vi "KF 연습 (A=eye(2)).vi"(2 "R":dbl[][](array[numeric])=[[1e-05, 0.0], [0.0, 1e-05]], 3 "Q":dbl[][](array[numeric])=[[0.001, 0.0], [0.0, 0.001]], 4 "Y_input":dbl format="%#.8g", 5 "X_input":dbl format="%#.8g") -> (0 "Y_Filtered":dbl format="%#.8g", 1 "X_Filtered":dbl format="%#.8g")   [LabVIEW 2016]
uses:
  <vilib>/imath/engines/lvmath2/RunTimeEngine/IndexRead/NIMS M(S).vi
  <instcachedir>/0/NIMS M(S)_B826C018497E4940AE96BD27B540B6FB.lvgen/NIMS M(S)_B826C018497E4940AE96BD27B540B6FB_000.vi
  <vilib>/imathl/engines/lvmath/Functions/Error Handling/Create Error.vi
  <vilib>/imath/engines/lvmath2/RunTimeEngine/ArithmeticOperatorToken/NIMS_ArithmeticOperator_multmx.vi
  <instcachedir>/0/NIMS_ArithmeticOperator_multmx_4A56FE5C615140CE835D4DB5891BF065.lvgen/NIMS_ArithmeticOperator_multmx_4A56FE5C615140CE835D4DB5891BF065_005.vi
  <instcachedir>/0/NIMS_ArithmeticOperator_multmx_4A56FE5C615140CE835D4DB5891BF065.lvgen/NIMS_ArithmeticOperator_multmx_4A56FE5C615140CE835D4DB5891BF065_006.vi
  <vilib>/imath/engines/lvmath2/RunTimeEngine/ArithmeticOperatorToken/NIMS_ArithmeticOperator_plus.vi
  <instcachedir>/0/NIMS_ArithmeticOperator_plus_0120E0498A0F4B4B9BDCAC2554767A4E.lvgen/NIMS_ArithmeticOperator_plus_0120E0498A0F4B4B9BDCAC2554767A4E_003.vi
  <vilib>/imath/engines/lvmath2/RunTimeEngine/ErrorHandling/NIMS_Create Error From Enums.vi
  <vilib>/imath/engines/lvmath2/RunTimeEngine/BuiltInFunctions/inv/NIMS_inv(GM).vi
  <instcachedir>/0/NIMS_inv(GM)_A6DF8FE880224208AACFE4CF9F659502.lvgen/NIMS_inv(GM)_A6DF8FE880224208AACFE4CF9F659502_000.vi
  <instcachedir>/0/NIMS_ArithmeticOperator_multmx_4A56FE5C615140CE835D4DB5891BF065.lvgen/NIMS_ArithmeticOperator_multmx_4A56FE5C615140CE835D4DB5891BF065_004.vi
  <vilib>/imath/engines/lvmath2/RunTimeEngine/ArithmeticOperatorToken/NIMS_ArithmeticOperator_multmx(M,CV).vi
  <instcachedir>/0/NIMS_ArithmeticOperator_multmx(M,CV)_EE734FC8520844C9A7CC1A67008668A3.lvgen/NIMS_ArithmeticOperator_multmx(M,CV)_EE734FC8520844C9A7CC1A67008668A3_000.vi
  <vilib>/imath/engines/lvmath2/RunTimeEngine/ArithmeticOperatorToken/NIMS_ArithmeticOperator_minus.vi
  <instcachedir>/0/NIMS_ArithmeticOperator_minus_E3B65B1D26A44BB184AFDC5B3F458E3D.lvgen/NIMS_ArithmeticOperator_minus_E3B65B1D26A44BB184AFDC5B3F458E3D_002.vi
  <vilib>/imath/engines/lvmath2/RunTimeEngine/NodeEndStatement/NIMS_NodeEndStatement_Output.vi
  <instcachedir>/0/NIMS_NodeEndStatement_Output_53EC0D466D134D7ABD903AC30B43404B.lvgen/NIMS_NodeEndStatement_Output_53EC0D466D134D7ABD903AC30B43404B_001.vi
  <instcachedir>/0/NIMS_NodeEndStatement_Output_53EC0D466D134D7ABD903AC30B43404B.lvgen/NIMS_NodeEndStatement_Output_53EC0D466D134D7ABD903AC30B43404B_002.vi
  <vilib>/imath/engines/lvmath2/RunTimeEngine/ErrorHandling/NIMS_Finalize Error.vi
panel:
  in  "P0":dbl[][](array[numeric])=[[1.0, 0.0], [0.0, 1.0]]
  out "K (Kalman Gain)":dbl[][](array[numeric])
  out "P (Covariance Matrix))":dbl[][](array[numeric])
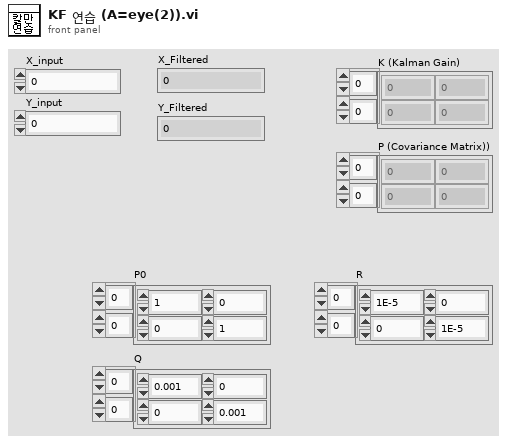
[diagram p1: front panel]
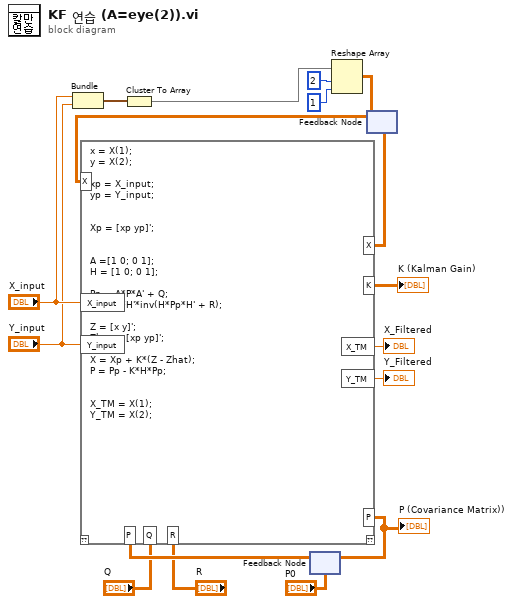
[diagram p0: block diagram]
diagram:
  n1 = Bundle("X_input"="X_input", "Y_input"="Y_input") -> (w3:cluster{"X_input":dbl, "Y_input":dbl})  [unwired: 1 in]
  n2 = Cluster To Array(cluster=w3) -> (array=w11:dbl[])
  n3 = feedback #1("P0") -> (w16:dbl[][])
  n4 = Reshape Array(w11, 2 ("차원 크기"), 1 ("차원 크기")) -> (w10:dbl[][])
  n5 = feedback #2(w10) -> (w15:dbl[][])
  n6 = mathscript code="x = X(1);\ny = X(2);\n\nxp = X_input;\nyp = Y_input;\n\n\nXp = [xp yp]';\n\n\nA =[1 0; 0 1];\nH = [1 0; 0 1];\n\nPp = A*P*A' + Q;\nK = Pp*H'*inv(H*Pp*H' + R);\n\nZ = [x y]';\nZhat = [xp yp]';\n\nX = Xp + K*(Z - Zhat);\nP = Pp - K*H*Pp;\n\n\nX_TM = X(1);\nY_TM = X(2);"("P"=w16, "Q"="Q", "R"="R", "X"=w15, "X_input"="X_input", "Y_input"="Y_input") -> ("X"=w14:dbl[][], "P"=w17:dbl[][], "K"=→"K (Kalman Gain)":dbl[][], "X_TM"=→"X_Filtered":dbl, "Y_TM"=→"Y_Filtered":dbl)  [unwired: 1 in, 1 out]
  "P (Covariance Matrix))" <- w17
  n7 = feedback-in #1(w17) -> ()
  n8 = feedback-in #2(w14) -> ()
